vi "01Foot.vi"() -> ()   [LabVIEW 2015]
uses:
  <vilib>/DAQmx/read.llb/DAQmx Read.vi
  <vilib>/DAQmx/read.llb/DAQmx Read (Digital 1D U8 1Chan NSamp).vi
  <vilib>/DAQmx/create/channels.llb/DAQmx Create Channel (DI-Digital Input).vi
  <vilib>/DAQmx/configure/timing.llb/DAQmx Timing (Sample Clock).vi
  <vilib>/DAQmx/miscellaneous.llb/DAQmx Fill In Error Info.vi
  <vilib>/Utility/file.llb/Write Delimited Spreadsheet (DBL).vi
panel:
  out "Array":dbl[](array[numeric])
  out "Waveform Graph":dbl[](graph)
  out "Waveform Graph 4":dbl[](graph)
  out "Waveform Graph 3":dbl[](graph)
  out "Waveform Graph 2":dbl[](graph)
  out "Waveform Graph 1":dbl[](graph)
  out "Array 5":u32[](array[numeric])
  out "data":u8[](array[numeric])
  in  "stop":bool
  out "ms elapsed":u32
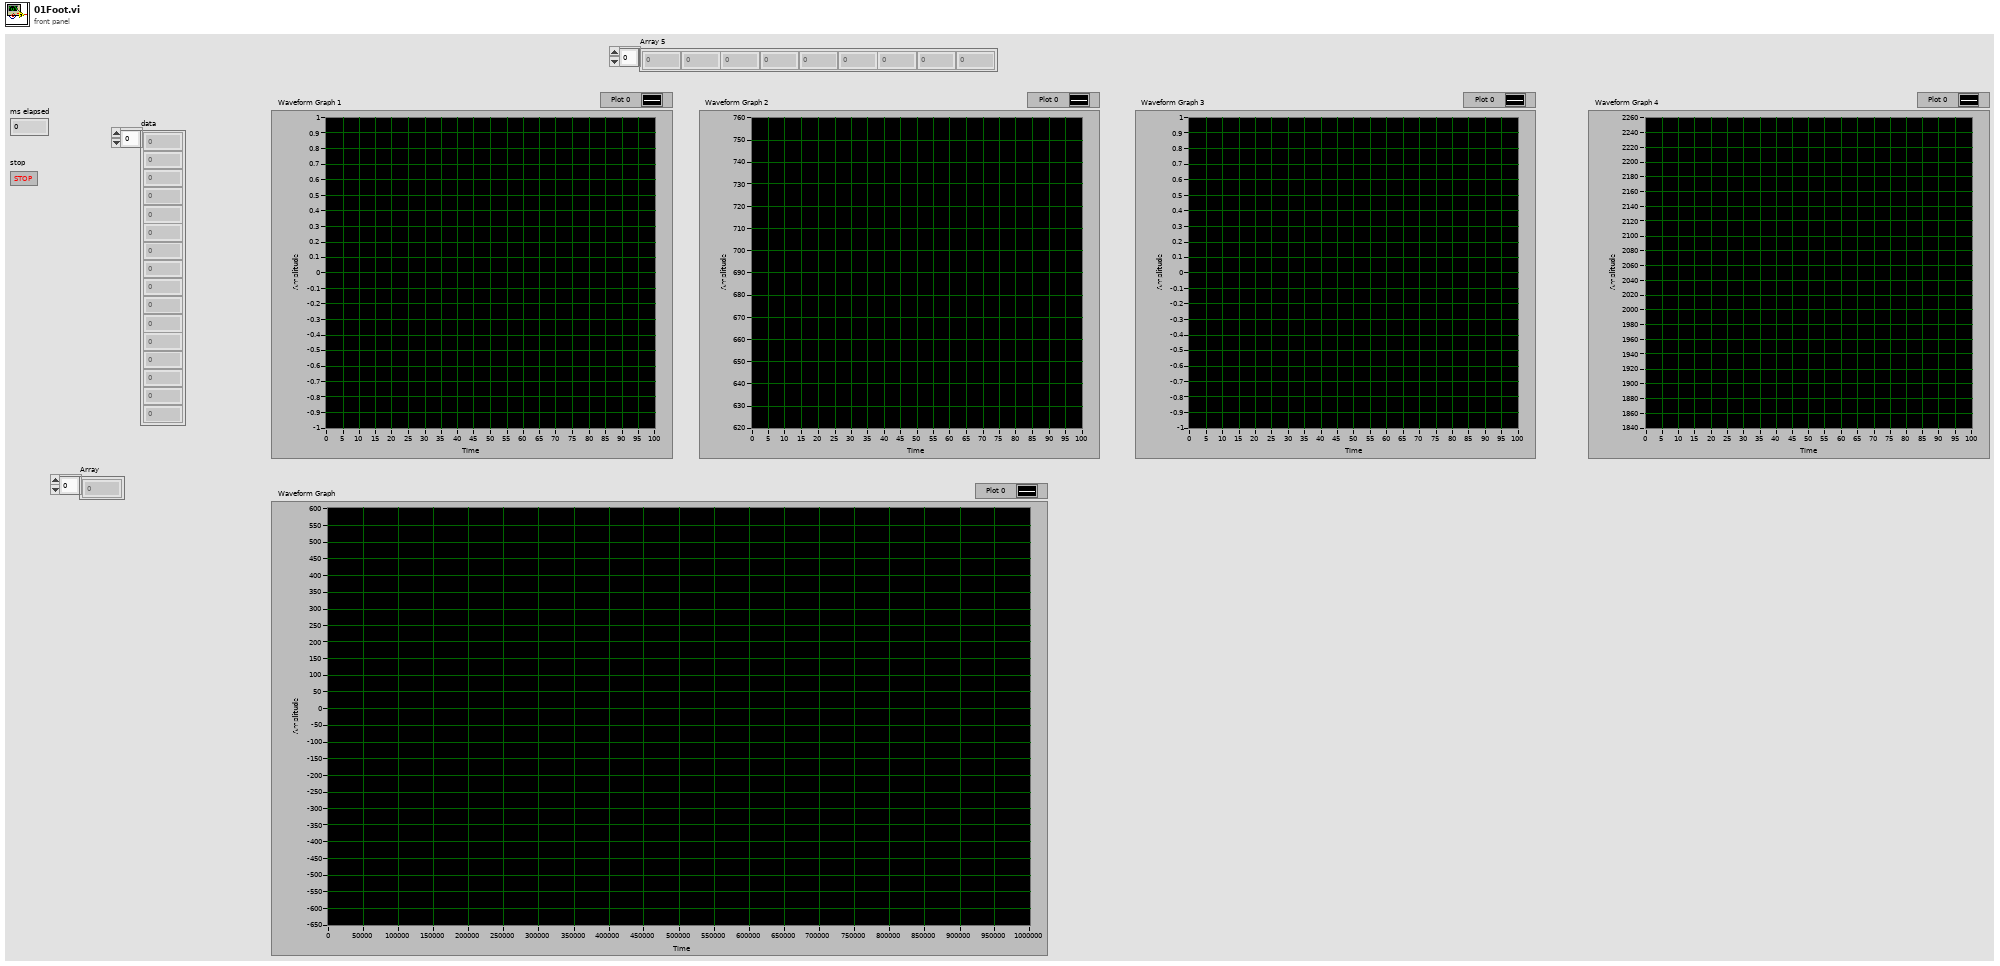
[diagram p1: front panel]
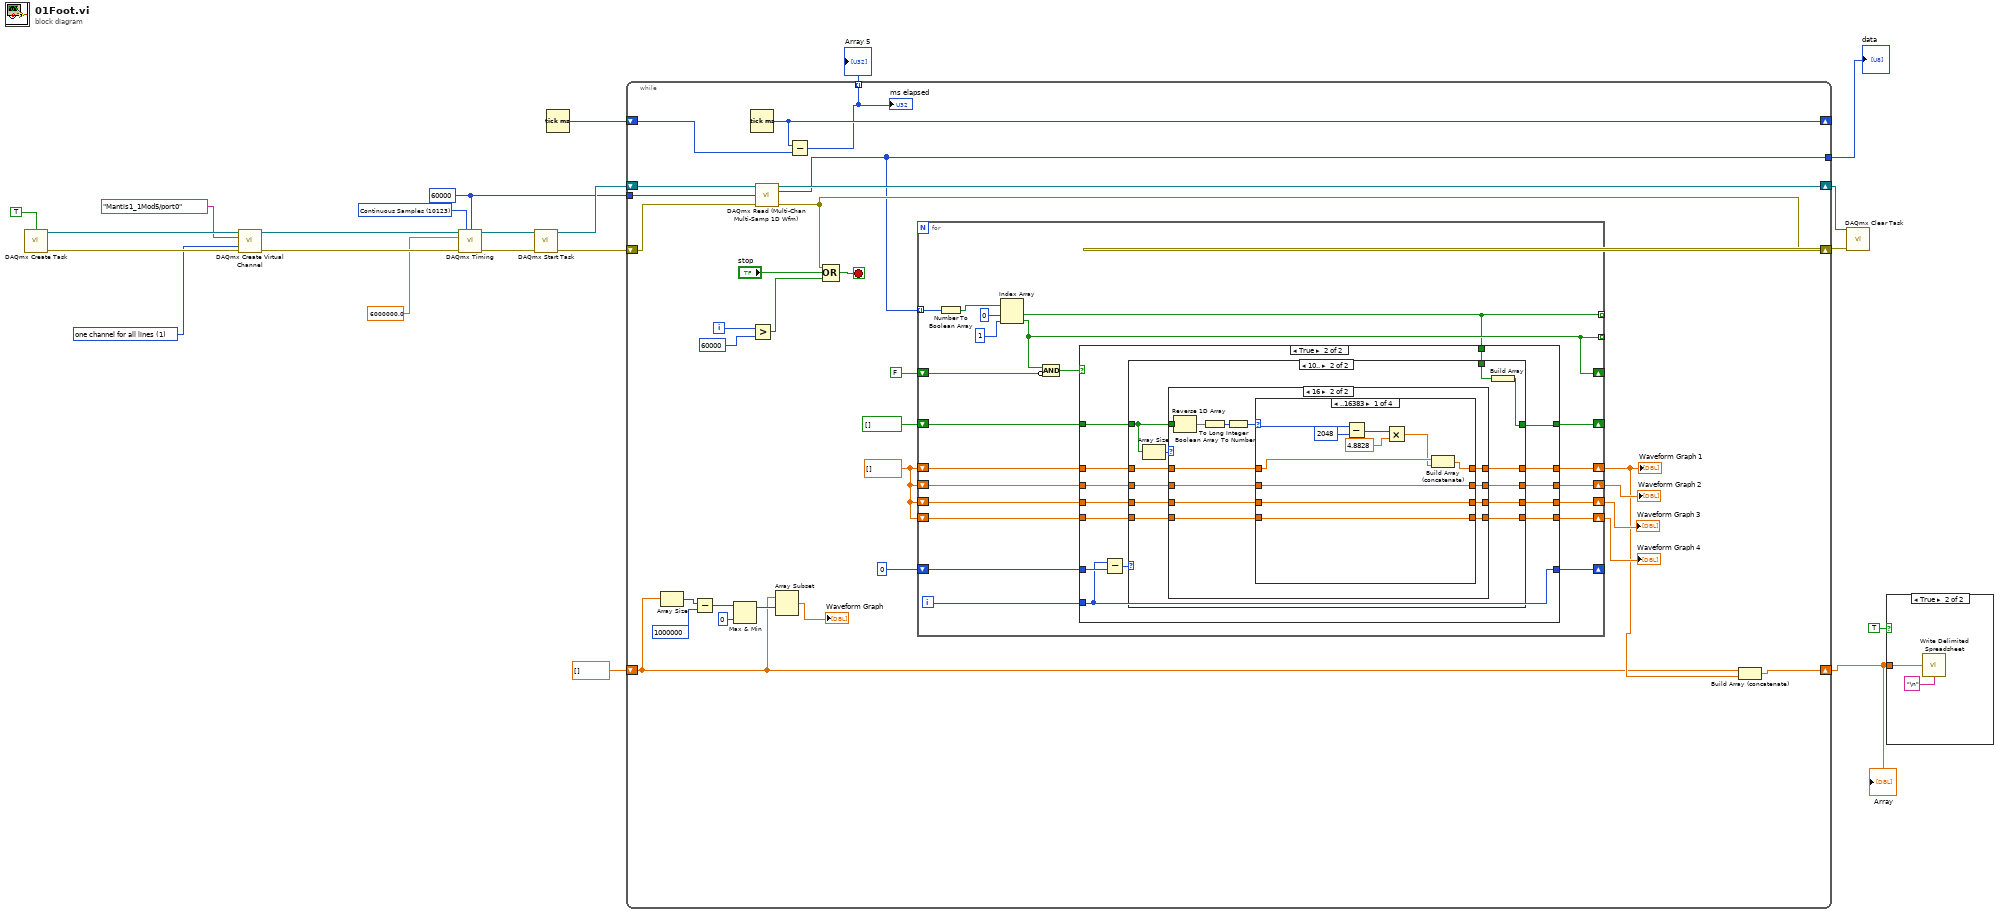
[diagram p0: block diagram]
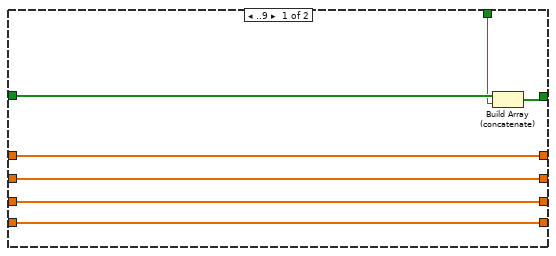
[diagram p4: hidden frame]
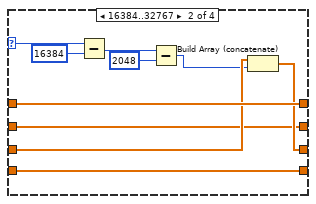
[diagram p6: hidden frame]
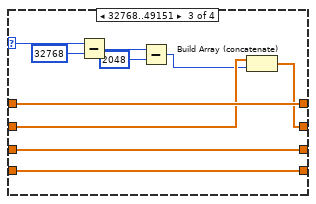
[diagram p7: hidden frame]
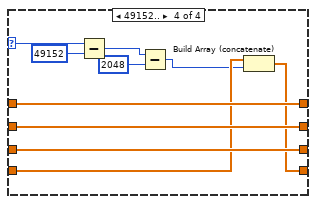
[diagram p8: hidden frame]
diagram:
  w9 = 60000 ("samples per channel")
  w10 = 10123 items=["Finite Samples"=10178, "Continuous Samples"=10123, "Hardware Timed Single Point"=12522] ("sample mode")
  w12 = 1 items=["one channel for each line", "one channel for all lines"] ("line grouping")
  n1 = call <vilib>:"DAQmx Create Task.vi"("auto cleanup"=TRUE) -> ("task out"=w19:refnum<k21>, "error out"=w18:errorcluster)  [unwired: 13 in]
  n2 = call-poly <vilib>:"DAQmx Create Virtual Channel.vi"("task in"=w19, "lines"=tag "Mantis1_1Mod5/port0", "line grouping"=w12, "error in"=w18) -> ("task out"=w21:refnum<k21>, "error out"=w20:errorcluster)  [unwired: 10 in]
  n3 = call-poly <vilib>:"DAQmx Timing.vi"("task/channels in"=w21, "sample mode"=w10, "samples per channel"=w9, "rate"=6000000.0, "error in"=w20) -> ("task out"=w17:refnum<k21>, "error out"=w16:errorcluster)  [unwired: 9 in]
  n4 = call <vilib>:"DAQmx Start Task.vi"("task/channels in"=w17, "error in"=w16) -> ("task out"=w14:refnum<k21>, "error out"=w15:errorcluster)  [unwired: 12 in]
  n5 = Tick Count (ms)() -> (millisecond timer value=w22:u32)
  n6 = while {
    shift-right: [w52] -> _
    shift-left: w22 -> [w51]
    shift-right: [w44] -> w6
    shift-left: w15 -> [w48]
    shift-right: [w47] -> w7
    shift-left: w14 -> [w50]
    tunnel: w9 -> [w49]
    tunnel: [w39] -> w5
    tunnel: [w40] -> w4 mode=indexing
    shift-right: [w37] -> w2
    shift-left: dbl[] [] -> [w27]
    i -> [w25]
    stop <- w46 stop-if-true
    w38 = dbl[] []
    n7 = Array Size(array=w27) -> (size(s)=w32:i32)
    n8 = Subtract(x=w32, y=1000000) -> (x-y=w30:i32)
    n9 = Max & Min(x=w30, y=0) -> (max(x,y)=w28:i32)  [unwired: 1 out]
    n10 = Tick Count (ms)() -> (millisecond timer value=w52:u32)
    n11 = Greater?(x=w25, y=60000) -> (0:w23:bool)
    n12 = call-poly "DAQmx Read (Multi-Chan Multi-Samp 1D Wfm).vi"("task/channels in"=w50, "number of samples per channel"=w49, "error in"=w48) -> ("task out"=w47:refnum<k21>, "data"=w39:u8[], "error out"=w44:errorcluster)  [unwired: 10 in]
    n13 = Array Subset(array=w27, index=w28) -> (→"Waveform Graph":dbl[])  [unwired: 1 in]
    n14 = Subtract(x=w52, y=w51) -> (x-y=w40:u32)
    "ms elapsed" <- w40
    n15 = Compound Arithmetic op=OR(w44, "stop", w23) -> (w46:bool)
    n16 = for {
      tunnel: w39 -> [w73] mode=indexing
      tunnel: [w63] -> _ mode=indexing
      tunnel: [w69] -> _ mode=indexing
      shift-right: [w69] -> _
      shift-left: FALSE -> [w68]
      shift-right: [w64] -> _
      shift-left: 0 -> [w65]
      shift-right: [w62] -> _
      shift-left: bool[] [] -> [w61]
      shift-right: [w60] -> w33
      shift-left: w38 -> [w59]
      shift-right: [w55] -> w36
      shift-left: w38 -> [w58]
      shift-right: [w54] -> w35
      shift-left: w38 -> [w57]
      shift-right: [w53] -> w34
      shift-left: w38 -> [w56]
      i -> [w66]
      n17 = Number To Boolean Array(number=w73) -> (Boolean array=w72:bool[])
      n18 = Index Array(array=w72, index #1=0 ("index"), index #2=1 ("index")) -> (element #1=w63:bool, element #2=w69:bool)
      n19 = Compound Arithmetic op=AND(w69, invert w68) -> (w67:bool)
      n20 = case shown="True" w67 {
        tunnel: w66 -> [_ w91]
        tunnel: w65 -> [w79 w93]
        tunnel: [w79 w91] -> w64
        tunnel: w63 -> [_ w90]
        tunnel: [w78 w88] -> w62
        tunnel: w61 -> [w78 w89]
        tunnel: [w77 w86] -> w60
        tunnel: w59 -> [w77 w87]
        tunnel: w58 -> [w76 w85]
        tunnel: w57 -> [w75 w84]
        tunnel: w56 -> [w74 w83]
        tunnel: [w76 w82] -> w55
        tunnel: [w75 w81] -> w54
        tunnel: [w74 w80] -> w53
        frame False {
        }
        frame True {
          n21 = Subtract(x=w91, y=w93) -> (x-y=w92:i32)
          n22 = case shown="10.." w92 {
            tunnel: w90 -> [w99 w111]
            tunnel: w89 -> [w100 w101]
            tunnel: [w98 w112] -> w88
            tunnel: w87 -> [w97 w110]
            tunnel: [w97 w106] -> w86
            tunnel: w85 -> [w96 w109]
            tunnel: w84 -> [w95 w108]
            tunnel: w83 -> [w94 w107]
            tunnel: [w96 w105] -> w82
            tunnel: [w95 w104] -> w81
            tunnel: [w94 w103] -> w80
            frame ..9 {
              n23 = Build Array (concatenate)(w100, w99) -> (w98:bool[])
            }
            frame 10.. {
              n24 = Array Size(array=w101) -> (size(s)=w102:i32)
              n25 = case shown="16" w102 {
                tunnel: w101 -> [_ w128]
                tunnel: w110 -> [w116 w126]
                tunnel: w109 -> [w115 w125]
                tunnel: w108 -> [w114 w124]
                tunnel: w107 -> [w113 w123]
                tunnel: [w116 w122] -> w106
                tunnel: [w115 w121] -> w105
                tunnel: [w114 w120] -> w104
                tunnel: [w113 w119] -> w103
                frame 0, Default {
                }
                frame 16 {
                  n26 = Reverse 1D Array(array=w128) -> (reversed array=w127:bool[])
                  n27 = Boolean Array To Number(Boolean array=w127) -> (number=w118:u32)
                  n28 = To Long Integer(number=w118) -> (32bit integer=w117:i32)
                  n29 = case shown="..16383" w117 {
                    selector: w117 -> [w133 w146 w156 w167]
                    tunnel: w126 -> [w138 w147 w157 w168]
                    tunnel: w125 -> [w136 w142 w153 w165]
                    tunnel: w124 -> [w135 w144 w154 w164]
                    tunnel: w123 -> [w134 w148 w158 w163]
                    tunnel: [w137 w147 w157 w168] -> w122
                    tunnel: [w136 w142 w152 w165] -> w121
                    tunnel: [w135 w143 w154 w164] -> w120
                    tunnel: [w134 w148 w158 w162] -> w119
                    frame ..16383 {
                      n30 = Subtract(x=w133, y=2048) -> (x-y=w131:i32)
                      n31 = Multiply(x=w131, y=4.8828) -> (x*y=w129:dbl)
                      n32 = Build Array (concatenate)(w138, w129) -> (w137:dbl[])
                    }
                    frame 16384..32767 {
                      n33 = Subtract(x=w146, y=16384) -> (x-y=w141:i32)
                      n34 = Subtract(x=w141, y=2048) -> (x-y=w139:i32)
                      n35 = Build Array (concatenate)(w144, w139) -> (w143:dbl[])
                    }
                    frame 32768..49151 {
                      n36 = Subtract(x=w156, y=32768) -> (x-y=w151:i32)
                      n37 = Subtract(x=w151, y=2048) -> (x-y=w149:i32)
                      n38 = Build Array (concatenate)(w153, w149) -> (w152:dbl[])
                    }
                    frame 49152.. {
                      n39 = Subtract(x=w167, y=49152) -> (x-y=w161:i32)
                      n40 = Subtract(x=w161, y=2048) -> (x-y=w159:i32)
                      n41 = Build Array (concatenate)(w163, w159) -> (w162:dbl[])
                    }
                  }
                }
              }
              n42 = Build Array(w111) -> (w112:bool[])
            }
          }
        }
      }
    }
    "Waveform Graph 1" <- w33
    "Waveform Graph 3" <- w35
    "Waveform Graph 4" <- w34
    "Waveform Graph 2" <- w36
    n43 = Build Array (concatenate)(w27, w33) -> (w37:dbl[])
  }
  "data" <- w5
  "Array 5" <- w4
  "Array" <- w2
  n44 = call <vilib>:"DAQmx Clear Task.vi"("task in"=w7, "error in"=w6) -> ()  [unwired: 13 in, 1 out]
  n45 = case shown="True" TRUE {
    tunnel: w2 -> [_ w170]
    frame False {
    }
    frame True {
      n46 = call-poly <vilib>:"Write Delimited Spreadsheet.vi"("1D data"=w170, "delimiter (\\t)"="\n" ("delimiter (\\t)")) -> ()  [unwired: 12 in, 2 out]
    }
  }
